vi "Lock Front Panel.vi"(8 "error in (no error)":errorcluster, 10 "Lock?":bool, 11 "2230G in":refnum<class "2230G.lvclass">) -> (0 "error out":errorcluster, 3 "2230G out":refnum<class "2230G.lvclass">)   [LabVIEW 2018, in "2230G.lvlib" / "2230G.lvclass"]
doc: "This VI allows the program to lock out front panel controls or unlock them."
uses:
  2230G.lvclass
  PPLs/Power Supply/Parent/Power_Supply.lvlibp/Power Supply.lvclass
  <instrlib>/Keithley KE22xx Series/Keithley KE22xx Series.lvlib
  C:/Projects/LabVIEW/PPLs/Power Supply/Parent/Power_Supply.lvlibp/Power Supply.lvclass
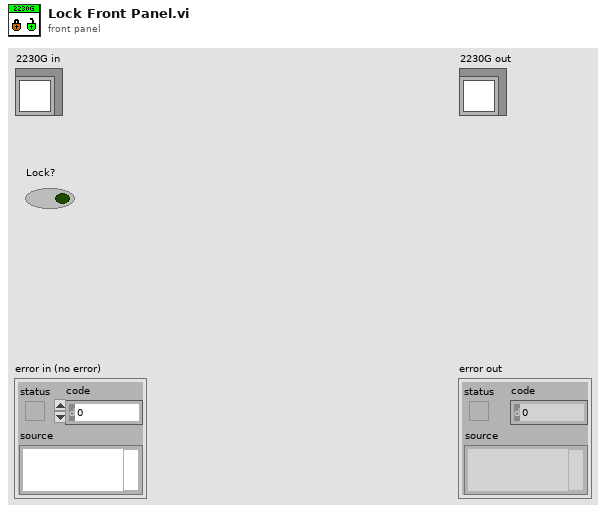
[diagram p1: front panel]
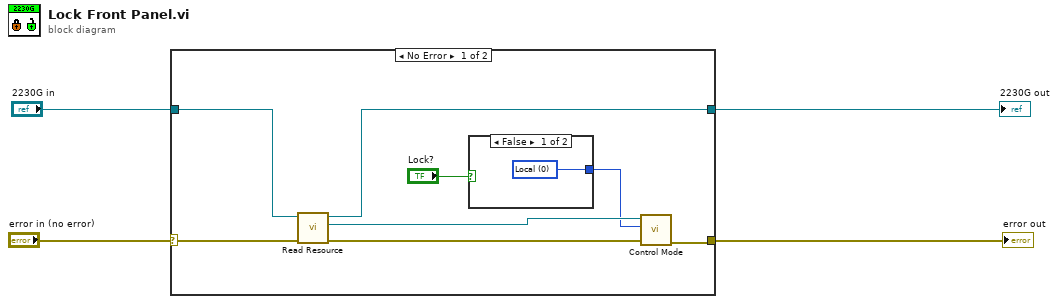
[diagram p0: block diagram]
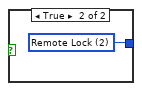
[diagram p2: hidden frame]
diagram:
  n1 = case shown="No Error" "error in (no error)" {
    selector: "error in (no error)" -> [w12 w16]
    tunnel: [w6 w16] -> w3
    tunnel: [w5 w15] -> w2
    tunnel: "2230G in" -> [w11 w15]
    frame No Error {
      n2 = call "Read Resource.vi"("error in"=w12, "Power Supply in"=w11) -> ("error out"=w9:errorcluster, "Resource"=w10:refnum<visa-resource-name>, "Power Supply out"=w5:refnum<class "2230G.lvclass">)  [unwired: 7 in]
      n3 = case shown="False" "Lock?" {
        tunnel: [w13 w14] -> w7
        frame False {
          w13 = u16 0 items=["Local", "Remote", "Remote Lock"] ("Control Mode (1: Remote)")
        }
        frame True {
          w14 = u16 2 items=["Local", "Remote", "Remote Lock"] ("Control Mode (1: Remote)")
        }
      }
      n4 = call <instrlib>:"Control Mode.vi"("error in (no error)"=w9, "Control Mode (1: Remote)"=w7, "VISA resource name"=w10) -> ("error out"=w6:errorcluster)  [unwired: 7 in, 1 out]
    }
    frame Error {
    }
  }
  "error out" <- w3
  "2230G out" <- w2
